vi "Tree Symble.vi"(8 "error in (no error)":errorcluster caption="Error In", 11 "Tree In":refnum<vi>) -> (0 "error out":errorcluster caption="Error Out", 3 "Tree Out":refnum<vi>)   [LabVIEW 2020]
panel:
  in  "Data Source List":string(tree)
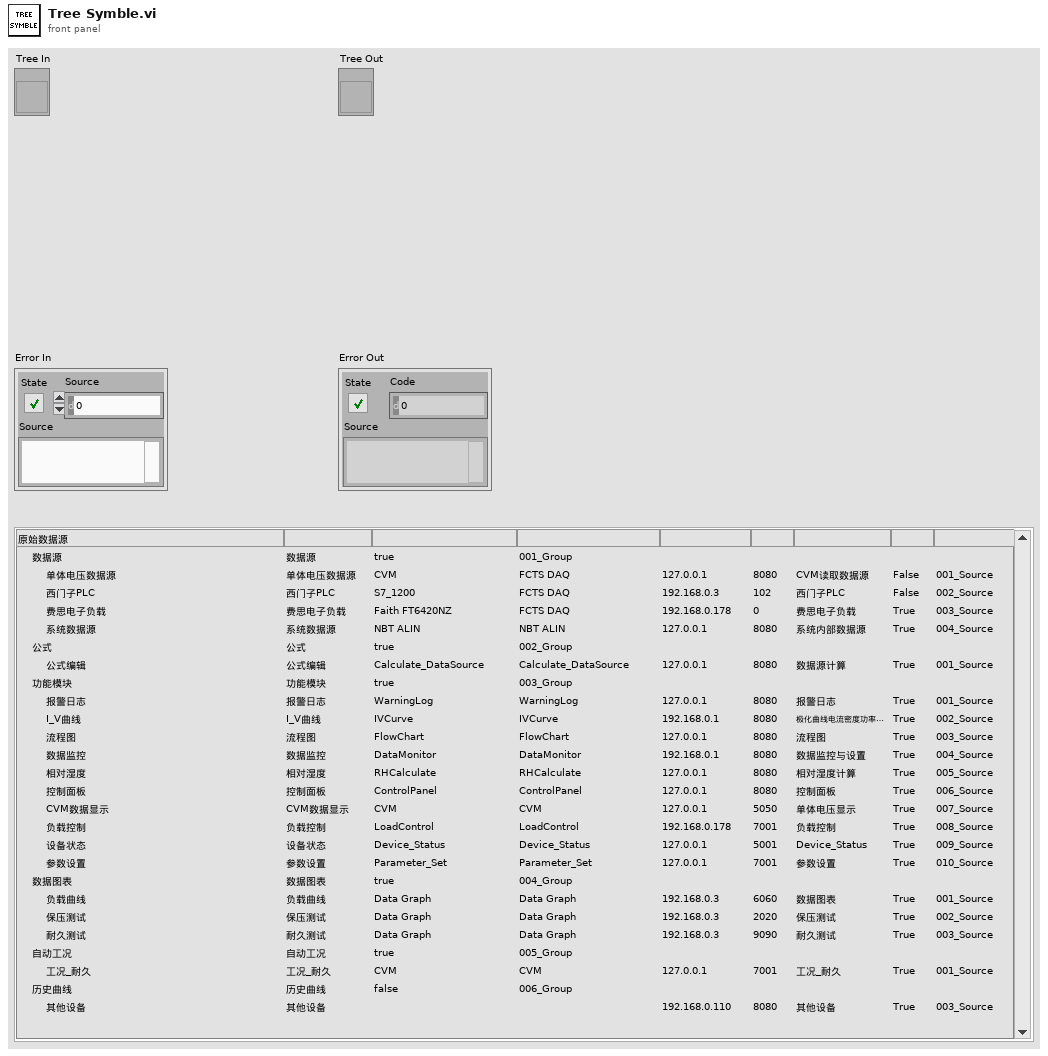
[diagram p1: front panel]
types:
  T1 = typedef "imagedata.ctl" = cluster{"image type":i32, "image depth":i32, "image":u8[], "mask":u8[], "colors":u32[], "Rectangle":cluster{"left":i16, "top":i16, "right":i16, "bottom":i16}}
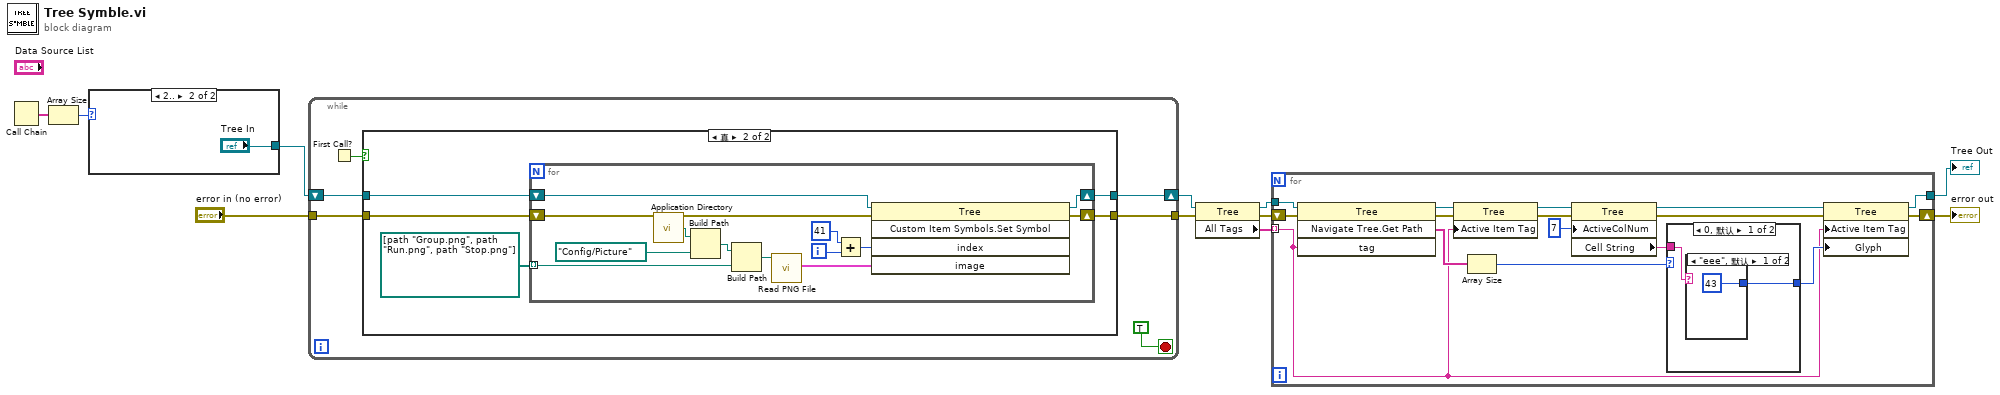
[diagram p0: block diagram]
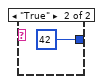
[diagram p3: hidden frame]
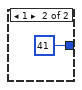
[diagram p4: hidden frame]
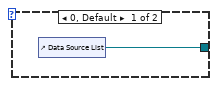
[diagram p5: hidden frame]
diagram:
  n1 = Call Chain() -> (call chain=w11:string[])
  n2 = Array Size(array=w11) -> (size(s)=w10:i32)
  n3 = case shown="2.." w10 {
    tunnel: [w12 "Tree In"] -> w5
    frame 0, Default {
      n4 = control-ref of="Data Source List"() -> (w12:refnum<vi>)
    }
    frame 2.. {
    }
  }
  n5 = while {
    shift-right: [w16] -> w4
    shift-left: w5 -> [w17]
    tunnel: [w15] -> w3
    tunnel: "error in (no error)" -> [w14]
    stop <- TRUE stop-if-true
    n6 = First Call?() -> (First Call?: T/F=w19:bool)
    n7 = case shown="真" w19 {
      tunnel: w17 -> [w21 w25]
      tunnel: [w21 w24] -> w16
      tunnel: [w20 w23] -> w15
      tunnel: w14 -> [w20 w22]
      frame False {
      }
      frame True {
        n8 = for {
          tunnel: path[] [path "Group.png", path "Run.png", path "Stop.png"] ("Picture Path") -> [w36] mode=indexing
          shift-right: [w29] -> w24
          shift-left: w25 -> [w30]
          shift-right: [w28] -> w23
          shift-left: w22 -> [w27]
          i -> [w33]
          n9 = call <vilib>:"Application Directory.vi"() -> ("Application Directory"=w39:path)
          n10 = Build Path(base path=w39, name or relative path=path "Config/Picture" ("路径")) -> (appended path=w37:path)
          n11 = Build Path(base path=w37, name or relative path=w36) -> (appended path=w35:path)
          n12 = call <vilib>:"Read PNG File.vi"("path to PNG file"=w35) -> ("image data"=w34:T1)  [unwired: 8 in, 2 out]
          n13 = Add(x=41, y=w33) -> (x+y=w31:i32)
          n14 = invoke class="Tree" method="Custom Item Symbols.Set Symbol"(reference=w30, error in=w27, "index"=w31, "image"=w34) -> (reference out=w29:refnum<vi>, error out=w28:errorcluster)  [unwired: 1 in, 3 out]
        }
      }
    }
  }
  n15 = property class="Tree"(reference=w4, error in=w3) -> (reference out=w7:refnum<vi>, error out=w2:errorcluster, "All Tags"=w6:string[])
  n16 = for {
    tunnel: [w54] -> w8
    tunnel: w7 -> [w53]
    shift-right: [w55] -> w9
    shift-left: w2 -> [w52]
    tunnel: w6 -> [w42] mode=indexing
    n17 = invoke class="Tree" method="Navigate Tree.Get Path"(reference=w53, error in=w52, "tag"=w42) -> (reference out=w44:refnum<vi>, error out=w41:errorcluster, "Navigate Tree:Get Path"=w48:string[])  [unwired: 1 in, 1 out]
    n18 = property class="Tree"(reference=w44, error in=w41, "Active Item Tag"=w42) -> (reference out=w43:refnum<vi>, error out=w40:errorcluster)
    n19 = Array Size(array=w48) -> (size(s)=w47:i32)
    n20 = property class="Tree"(reference=w43, error in=w40, "ActiveColNum"=7 ("活动单元格:活动列数")) -> (reference out=w51:refnum<vi>, error out=w49:errorcluster, "Cell String"=w45:string)
    n21 = case shown="0, 默认" w47 {
      tunnel: [w56 41 ("x")] -> w46
      tunnel: w45 -> [w57 _]
      frame 0, Default {
        n22 = case shown="\"eee\", 默认" w57 {
          tunnel: [43 ("x") 42 ("x")] -> w56
          frame "eee", Default {
          }
          frame "True" {
          }
        }
      }
      frame 1 {
      }
    }
    n23 = property class="Tree"(reference=w51, error in=w49, "Active Item Tag"=w42, "Glyph"=w46) -> (reference out=w54:refnum<vi>, error out=w55:errorcluster)
  }
  "error out" <- w9
  "Tree Out" <- w8
